vi "ROI_Analysis.vi"(8 "error in (no error)":errorcluster, 9 "Valid ROI":bool, 10 "ROI":T1 {"Contours"."Type" items=["No Selection", "Point", "Line", "Rectangle", "Oval", "Polygon", "Freehand Region", "Annulus", "Unused2", "Unused3", "Broken Line", "Freehand Line", "Rotated Rectangle"]}, 11 "Image In":T2) -> (0 "error out":errorcluster, 2 "ROI Results":dbl, 3 "ROI Snippet Out":T2)   [LabVIEW 2014]
uses:
  <vilib>/vision/Image Controls.llb/IMAQ Image.ctl
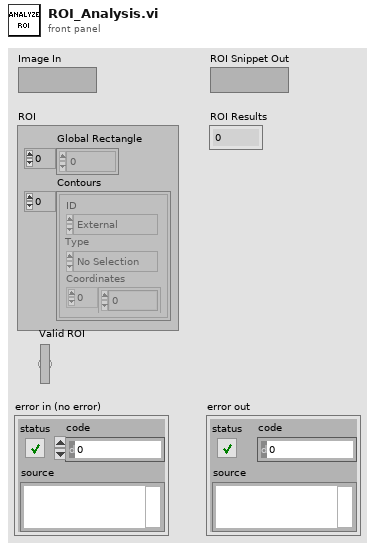
[diagram p1: front panel]
types:
  T1 = typedef "ROI Descriptor" = cluster{"Global Rectangle":i32[], "Contours":cluster{"ID":enum32{"External", "Internal"}, "Type":u32, "Coordinates":i32[]}[]}
  T2 = typedef "IMAQ Image.ctl" = refnum<image>
  T3 = typedef "Image Type" = u32
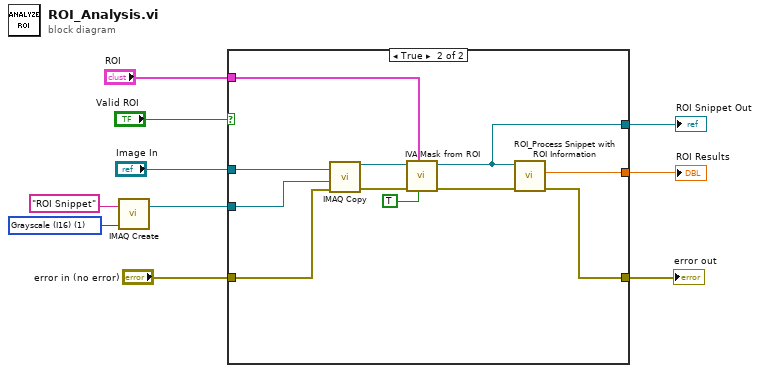
[diagram p0: block diagram]
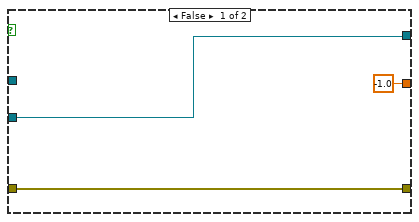
[diagram p2: hidden frame]
diagram:
  w9 = T3 1 items=["Grayscale (U8)", "Grayscale (I16)", "Grayscale (SGL)", "Complex (CSG)", "RGB (U32)", "HSL (U32)", "RGB (U64)", "Grayscale (U16)"] ("Image Type")
  n1 = call "IMAQ Create"("Image Name"="ROI Snippet", "Image Type"=w9) -> ("New Image"=w10:T2)  [unwired: 2 in, 2 out]
  n2 = case shown="True" "Valid ROI" {
    tunnel: w10 -> [w11 w24]
    tunnel: [w11 w23] -> w7
    tunnel: "Image In" -> [_ w22]
    tunnel: "error in (no error)" -> [w13 w21]
    tunnel: [w13 w18] -> w4
    tunnel: [-1.0 ("ROI Information") w17] -> w3
    tunnel: "ROI" -> [_ w15]
    frame False {
    }
    frame True {
      n3 = call "IMAQ Copy"("error in (no error)"=w21, "Image Dst"=w24, "Image Src"=w22) -> ("error out"=w19:errorcluster, "Image Dst Out"=w20:T2)  [unwired: 3 in]
      n4 = call <vilib>:"IVA Mask from ROI.vi"("Shrink"=TRUE, "ROI Descriptor"=w15, "error in (no error)"=w19, "Image Src"=w20) -> ("error out"=w14:errorcluster, "Image Out"=w23:T2)  [unwired: 1 in, 5 out]
      n5 = call "ROI_Process Snippet with ROI Information.vi"("error in (no error)"=w14, "ROI Snippet"=w23) -> ("error out"=w18:errorcluster, "ROI Information"=w17:dbl)  [unwired: 8 in]
    }
  }
  "ROI Snippet Out" <- w7
  "error out" <- w4
  "ROI Results" <- w3
